vi "Configure Sequencer List Frequency.vi"(7 "Frequency (1.2GHz)":dbl=1200000000.0 format="%#.9p", 8 "error in (no error)":errorcluster, 9 "Index (0)":i32, 10 "Instance (1)":i32=1, 11 "VISA resource name":refnum<visa-resource-name>) -> (0 "error out":errorcluster, 3 "VISA resource name out":refnum<visa-resource-name>)   [LabVIEW 2015, in "Rohde&Schwarz CMXP GPRF.lvlib"]
doc: "Defines the RF generator frequency for the sequencer list entry with the selected Index.\n\nAttribute:\nRSCMXPGPRF_ATTR_SEQUENCER_LIST_FREQUENCY\n\nRemote-control command:\nSOURce:GPRF:GEN<i>:SEQuencer:LIST:FREQuency"
uses:
  <instrlib>/Rohde&Schwarz CMXP GPRF/Rohde&Schwarz CMXP GPRF.lvlib
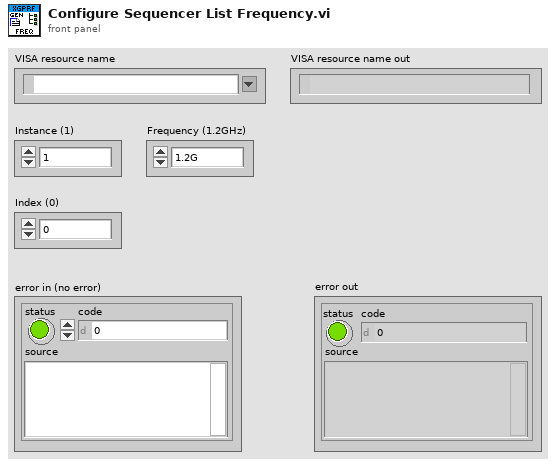
[diagram p1: front panel]
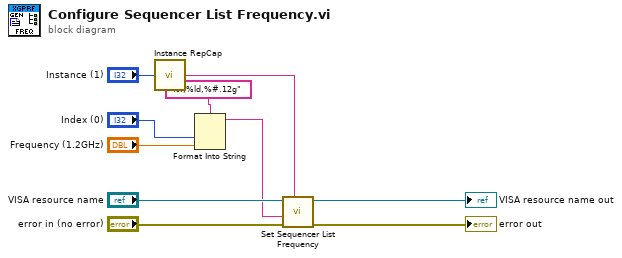
[diagram p0: block diagram]
diagram:
  n1 = call <instrlib>:"Instance RepCap.vi"("Instance in"="Instance (1)") -> ("Instance out"=w5:string)
  n2 = Format Into String(format string="%.;%ld,%#.12g", "Index (0)", "Frequency (1.2GHz)") -> (resulting string=w1:string)  [unwired: 2 in, 1 out]
  n3 = call "Set Sequencer List Frequency"("Repeated Capabilities"=w5, "error in (no error)"="error in (no error)", "Sequencer List Frequency ()"=w1, "instrument handle"="VISA resource name") -> ("error out"=→"error out":errorcluster, "instrument handle out"=→"VISA resource name out":refnum<visa-resource-name>)  [unwired: 6 in]
